vi "simu col types.vi"(10 "ring?":bool) -> (2 "ColTypes[ ]":T1[](array[typedef]))   [LabVIEW 2016]
uses:
  HardWare/Ctrls/HardWare _ Channel Configurations PopUp Type.ctl
  ToolKit/Popup/Private/Ctrls/POP_Data Type.ctl
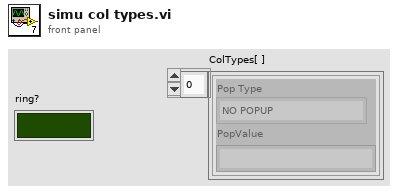
[diagram p1: front panel]
types:
  T1 = typedef "HardWare _ Channel Configurations PopUp Type.ctl" = cluster{"Pop Type":T2, "PopValue":string}
  T2 = typedef "POP_Data Type.ctl" = enum16{"NO POPUP", "Unkown", "String", "Integer", "Float", "Color", "Boolean", "Ring", "Captioned String", "Captioned Integer", "Button Color", "2 Int Cluster", "4 Int Cluster", "6-Dbl Cluster", "Path", "Combox", "Time", "ShotCut String"}
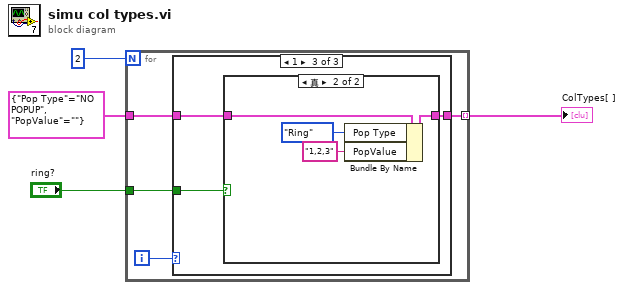
[diagram p0: block diagram]
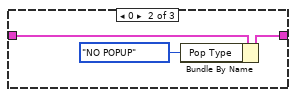
[diagram p3: hidden frame]
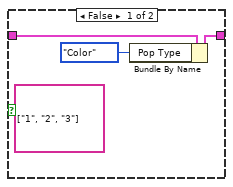
[diagram p4: hidden frame]
diagram:
  n1 = for {
    N: 2 -> [_]
    tunnel: T1 {"Pop Type"=enum."NO POPUP", "PopValue"=""} ("ColType") -> [w7]
    tunnel: [w6] -> w2 mode=indexing
    tunnel: "ring?" -> [w5]
    i -> [w8]
    n2 = case shown="1" w8 {
      tunnel: w7 -> [w9 w12 w15]
      tunnel: [w9 w11 w14] -> w6
      tunnel: w5 -> [_ _ w13]
      frame Default {
      }
      frame 0 {
        n3 = Bundle By Name(cluster=w12, "Pop Type"=POP_Data_Type."NO POPUP" ("Prop Type")) -> (w11:T1)
      }
      frame 1 {
        n4 = case shown="真" w13 {
          tunnel: w15 -> [w18 w22]
          tunnel: [w17 w21] -> w14
          frame False {
            (unwired) string[] ["1", "2", "3"]
            n5 = Bundle By Name(cluster=w18, "Pop Type"=POP_Data_Type."Color" ("Prop Type")) -> (w17:T1)
          }
          frame True {
            n6 = Bundle By Name(cluster=w22, "Pop Type"=POP_Data_Type."Ring" ("Prop Type"), "PopValue"="1,2,3") -> (w21:T1)
          }
        }
      }
    }
  }
  "ColTypes[ ]" <- w2
